vi "AnalyseLiveLV.vi"(8 "error in (no error)":errorcluster, 10 "ImageData":T3, 11 "FluorescenceLiveAnalyser in":refnum<class "FluorescenceLiveAnalyser.lvclass">) -> (0 "error out":errorcluster, 3 "FluorescenceLiveAnalyser out":refnum<class "FluorescenceLiveAnalyser.lvclass">)   [LabVIEW 2011, in "Tools.lvlib" / "Imaging.lvlib" / "FluorescenceLiveAnalyser.lvclass"]
uses:
  FluorescenceLiveAnalyser.lvclass
  <vilib>/Analysis/NI_AALBase.lvlib
  ImageAnalyser.lvclass
  Imaging.lvlib
panel:
  in  "threshold":dbl=0.3
  in  "exposuretime":dbl=0.003
  in  "Settings":T1={"Objects"=0, "Threshold"=0, "Reject Border"=TRUE, "Fill Holes"=FALSE, "Min Object Size"=TRUE, "Min Size"=1000, "Max Object Size"=FALSE, "Max Size"=1500000, "Show Search Area"=TRUE, "Show Center"=TRUE, "Show Bounding Box"=TRUE} {"Objects" items=["Bright Objects", "Dark Objects"]}
  in  "detuning MHz":dbl=-12.0
  out "Image":T2(plugin-control)
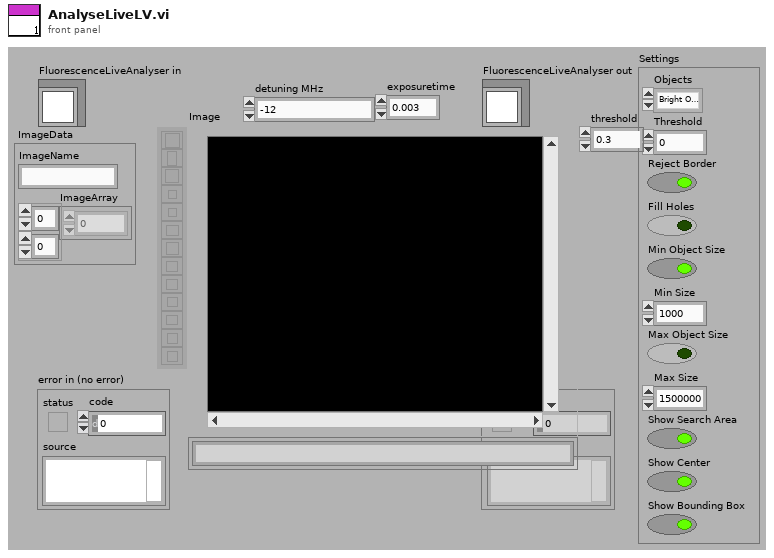
[diagram p1: front panel]
types:
  T1 = cluster{"Objects":u16, "Threshold":i32, "Reject Border":bool, "Fill Holes":bool, "Min Object Size":bool, "Min Size":i32, "Max Object Size":bool, "Max Size":i32, "Show Search Area":bool, "Show Center":bool, "Show Bounding Box":bool}
  T2 = typedef "IMAQ Image.ctl" = refnum<image>
  T3 = cluster{"ImageName":string, "ImageArray":sgl[][]}
  T4 = typedef "IMAQ Rectangle" = cluster{"Left":i32, "Top":i32, "Right":i32, "Bottom":i32, "Rotation":dbl}
  T5 = cluster{"Name":string, "Results":dbl[], "AnalysisType":string}
  T6 = typedef "Image Type" = u32
  T7 = cluster{"Left":i32, "Top":i32, "Right":i32, "Bottom":i32}
  T8 = cluster{"Object Center":cluster{"X":sgl, "Y":sgl}, "Bounding Box":cluster{"X Left":i32, "Y Top":i32, "X Right":i32, "Y Bottom":i32}, "Area":sgl, "Orientation":sgl, "Aspect Ratio":sgl, "Nb Holes":i32}[]
  T9 = cluster{"Object Center":cluster{"X":sgl, "Y":sgl}, "Bounding Box":cluster{"X Left":i32, "Y Top":i32, "X Right":i32, "Y Bottom":i32}, "Area":sgl, "Orientation":sgl, "Aspect Ratio":sgl, "Nb Holes":i32}
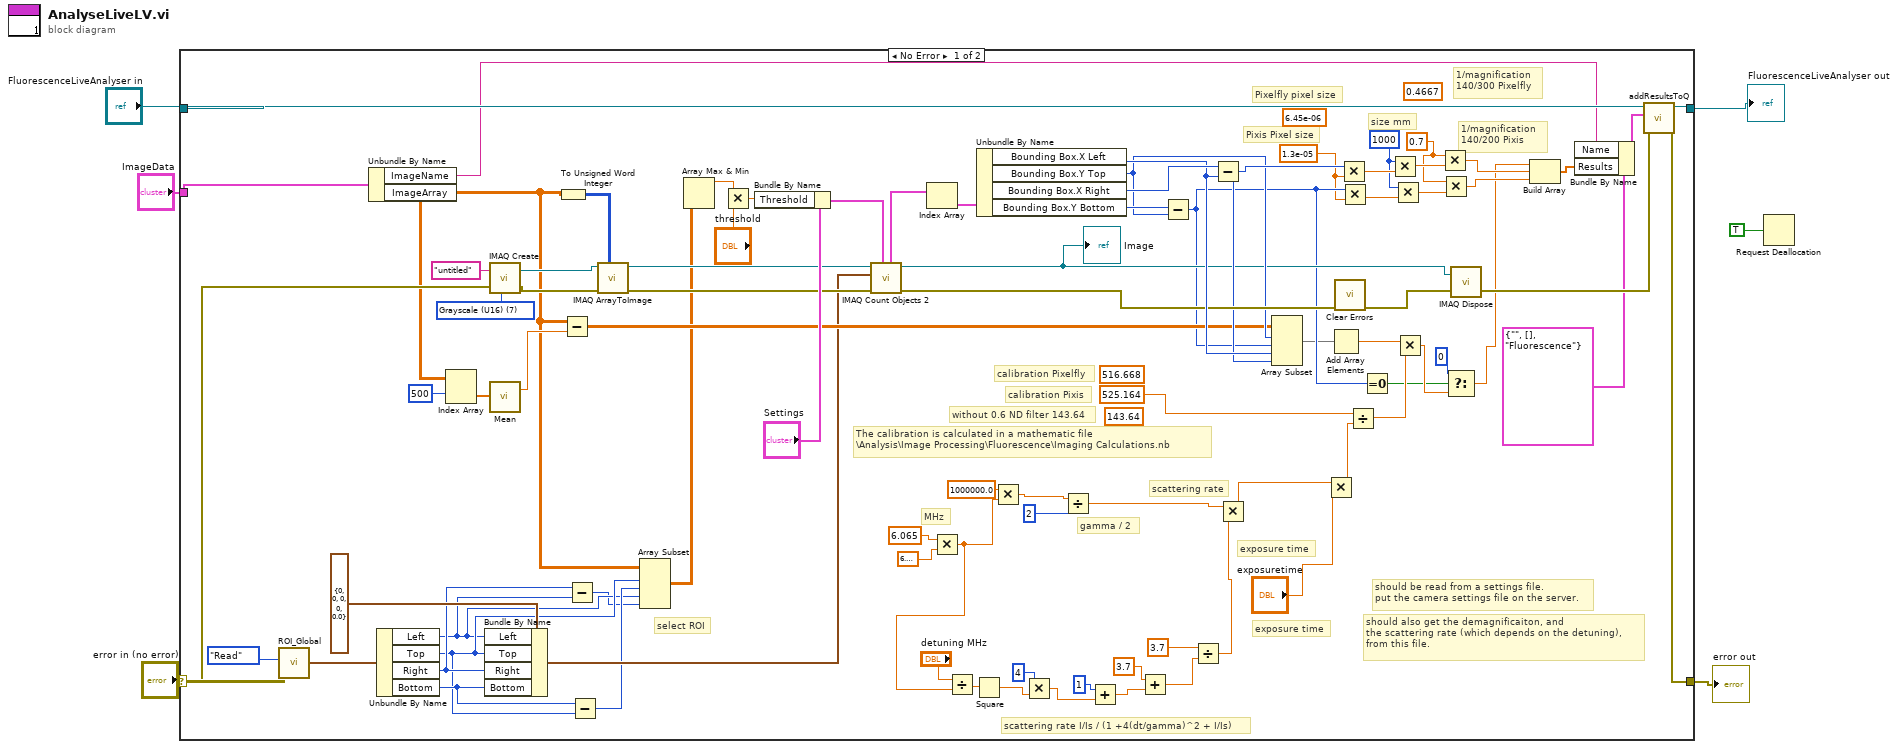
[diagram p0: block diagram]
diagram:
  n1 = case shown="No Error" "error in (no error)" {
    selector: "error in (no error)" -> [w76 w95]
    tunnel: [w66 w95] -> w5
    tunnel: [w68 w94] -> w1
    tunnel: "FluorescenceLiveAnalyser in" -> [w67 w94]
    tunnel: "ImageData" -> [w93 _]
    frame No Error {
      (unwired) 143.64
      (unwired) 0.4667
      (unwired) 6.45e-06
      (unwired) 516.668
      w10 = 0.7
      w61 = 1000
      w11 = 1.3e-05
      w78 = T6 7 items=["Grayscale (U8)", "Grayscale (I16)", "Grayscale (SGL)", "Complex (CSG)", "RGB (U32)", "HSL (U32)", "RGB (U64)", "Grayscale (U16)"] ("Image Type")
      # "select ROI"
      # "1/magnification\n140/300 Pixelfly"
      # "Pixelfly pixel size"
      # "calibration Pixelfly"
      # "gamma / 2"
      # "scattering rate I/Is / (1 +4(dt/gamma)^2 + I/Is)"
      # "MHz"
      # "exposure time"
      # "scattering rate"
      # "without 0.6 ND filter 143.64"
      # "Pixis Pixel size"
      # "should also get the demagnificaiton, and\nthe scattering rate (which depends on the detuning),\nfrom this file."
      # "should be read from a settings file.\nput the camera settings file on the server."
      # "The calibration is calculated in a mathematic file\n\\Analysis\\Image Processing\\Fluorescence\\Imaging Calculations.nb"
      # "1/magnification\n140/200 Pixis"
      # "size mm"
      # "exposure time"
      # "calibration Pixis"
      n2 = call "ROI_Global.vi"("Action"=enum16{"Write", "Read"}."Read") -> ("ROI"=w40:T7)  [unwired: 10 in]
      n3 = Unbundle By Name(w93) -> ("ImageName"=w55:string, "ImageArray"=w7:sgl[][])
      n4 = Unbundle By Name(w40) -> ("Left"=w14:i32, "Top"=w16:i32, "Right"=w17:i32, "Bottom"=w18:i32)
      n5 = Index Array(array=w7, index (row)=500) -> (element=w73:sgl[])  [unwired: 1 in]
      n6 = Bundle By Name(cluster=T4 {"Left"=0, "Top"=0, "Right"=0, "Bottom"=0, "Rotation"=0.0} ("Search Rect (entire image)"), "Left"=w14, "Top"=w16, "Right"=w17, "Bottom"=w18) -> (w39:T4)
      n7 = call "IMAQ Create"("Image Name"="untitled", "Image Type"=w78, "error in (no error)"=w76) -> ("New Image"=w92:T2, "error out"=w91:errorcluster)  [unwired: 2 in]
      n8 = call <vilib>:"Mean.vi"("X"=w73) -> ("mean"=w46:dbl)  [unwired: 1 out]
      n9 = To Unsigned Word Integer(number=w7) -> (unsigned 16bit integer=w8:u16[][])
      n10 = Subtract(x=w7, y=w46) -> (x-y=w50:dbl[][])
      n11 = Subtract(x=w17, y=w14) -> (x-y=w13:i32)
      n12 = Subtract(x=w18, y=w16) -> (x-y=w15:i32)
      n13 = call "IMAQ ArrayToImage"("Image Pixels (U16)"=w8, "error in (no error)"=w91, "Image"=w92) -> ("error out"=w83:errorcluster, "Image Out"=w84:T2)  [unwired: 7 in]
      n14 = Array Subset(array=w7, index (row)=w16, length (row)=w15, index (col)=w14, length (col)=w13) -> (w12:sgl[][])
      n15 = Array Max & Min(array=w12) -> (max value=w87:sgl)  [unwired: 3 out]
      n16 = Multiply(x=w87, y="threshold") -> (x*y=w88:dbl)
      n17 = Bundle By Name(cluster="Settings", "Threshold"=w88) -> (w85:T1)
      n18 = call "IMAQ Count Objects 2"("Settings"=w85, "error in (no error)"=w83, "Search Rect (entire image)"=w39, "Image"=w84) -> ("error out"=w77:errorcluster, "Image Out"=w60:T2, "Objects"=w82:T8)  [unwired: 3 in, 2 out]
      "Image" <- w60
      n19 = Index Array(array=w82) -> (element=w81:T9)  [unwired: 1 in]
      n20 = Multiply(x=6.065, y=6.283185307179586) -> (x*y=w29:dbl)
      n21 = Divide(x="detuning MHz", y=w29) -> (x/y=w28:dbl)
      n22 = Square(x=w28) -> (x^2=w27:dbl)
      n23 = Unbundle By Name(w81) -> ("Bounding Box.X Left"=w79:i32, "Bounding Box.Y Top"=w64:i32, "Bounding Box.X Right"=w80:i32, "Bounding Box.Y Bottom"=w65:i32)
      n24 = Multiply(x=1000000.0, y=w29) -> (x*y=w35:dbl)
      n25 = Multiply(x=4, y=w27) -> (x*y=w26:dbl)
      n26 = Divide(x=w35, y=2) -> (x/y=w22:dbl)
      n27 = Add(x=1, y=w26) -> (x+y=w25:dbl)
      n28 = Add(x=3.7, y=w25) -> (x+y=w23:dbl)
      n29 = Subtract(x=w65, y=w64) -> (x-y=w45:i32)
      n30 = Divide(x=3.7, y=w23) -> (x/y=w21:dbl)
      n31 = Subtract(x=w80, y=w79) -> (x-y=w75:i32)
      n32 = Multiply(x=w22, y=w21) -> (x*y=w20:dbl)
      n33 = Array Subset(array=w50, index (row)=w64, length (row)=w45, index (col)=w79, length (col)=w75) -> (w43:dbl[][])
      n34 = Multiply(x=w20, y="exposuretime") -> (x*y=w72:dbl)
      n35 = Add Array Elements(numeric array=w43) -> (sum=w70:dbl)
      n36 = call <vilib>:"Clear Errors.vi"("error in (no error)"=w77) -> ("error out"=w59:errorcluster)  [unwired: 6 in]
      n37 = Multiply(x=w75, y=w11) -> (x*y=w63:dbl)
      n38 = Multiply(x=w45, y=w11) -> (x*y=w62:dbl)
      n39 = Divide(x=525.164, y=w72) -> (x/y=w69:dbl)
      n40 = Equal To 0?(x=w45) -> (x = 0?=w44:bool)
      n41 = Multiply(x=w61, y=w63) -> (x*y=w19:dbl)
      n42 = Multiply(x=w61, y=w62) -> (x*y=w53:dbl)
      n43 = Multiply(x=w70, y=w69) -> (x*y=w48:dbl)
      n44 = Multiply(x=w10, y=w19) -> (x*y=w52:dbl)
      n45 = Multiply(x=w10, y=w53) -> (x*y=w51:dbl)
      n46 = Select(t=0, s=w44, f=w48) -> (s? t:f=w47:dbl)
      n47 = call "IMAQ Dispose"("Image"=w60, "error in (no error)"=w59) -> ("error out"=w58:errorcluster)  [unwired: 4 in]
      n48 = Build Array(w47, w52, w51) -> (w56:dbl[])
      n49 = Bundle By Name(cluster=T5 {"Name"="", "Results"=[], "AnalysisType"="Fluorescence"} ("output cluster"), "Name"=w55, "Results"=w56) -> (w54:T5)
      n50 = call "addResultsToQ.vi"("error in (no error)"=w58, "Results"=w54, "ImageAnalyser in"=w67) -> ("error out"=w66:errorcluster, "ImageAnalyser out"=w68:refnum<class "FluorescenceLiveAnalyser.lvclass">)  [unwired: 7 in]
    }
    frame Error {
    }
  }
  "error out" <- w5
  "FluorescenceLiveAnalyser out" <- w1
  n51 = Request Deallocation(TRUE ("flag")) -> ()
